vi "advent_4._bvi.vi"() -> ()   [LabVIEW 2021]
uses:
  <vilib>/Utility/file.llb/Read Delimited Spreadsheet (string).vi
  <vilib>/Utility/file.llb/Read Delimited Spreadsheet (I64).vi
panel:
  out "Array 3":i32[](array[numeric])
  out "array w/ subset deleted":string[][](array[string])
  out "all rows 2":string[][](array[string])
  out "final value":i32
  out "last number called":u8
  out "sum of unmarked":i32
  out "all rows":string[](array[string])
  out "size(s)":i32
  out "final bingo call":i32
  out "Book Number":i32
  out "Array":bool[][][](array[boolean])
  out "card values":i32[][](array[numeric])
  out "card":bool[][](array[boolean])
  out "initialized array":bool[][][](array[boolean])
  out "Array 2":i32[][][](array[numeric])
  out "subarray":string[](array[string])
  out "first row":i64[](array[numeric])
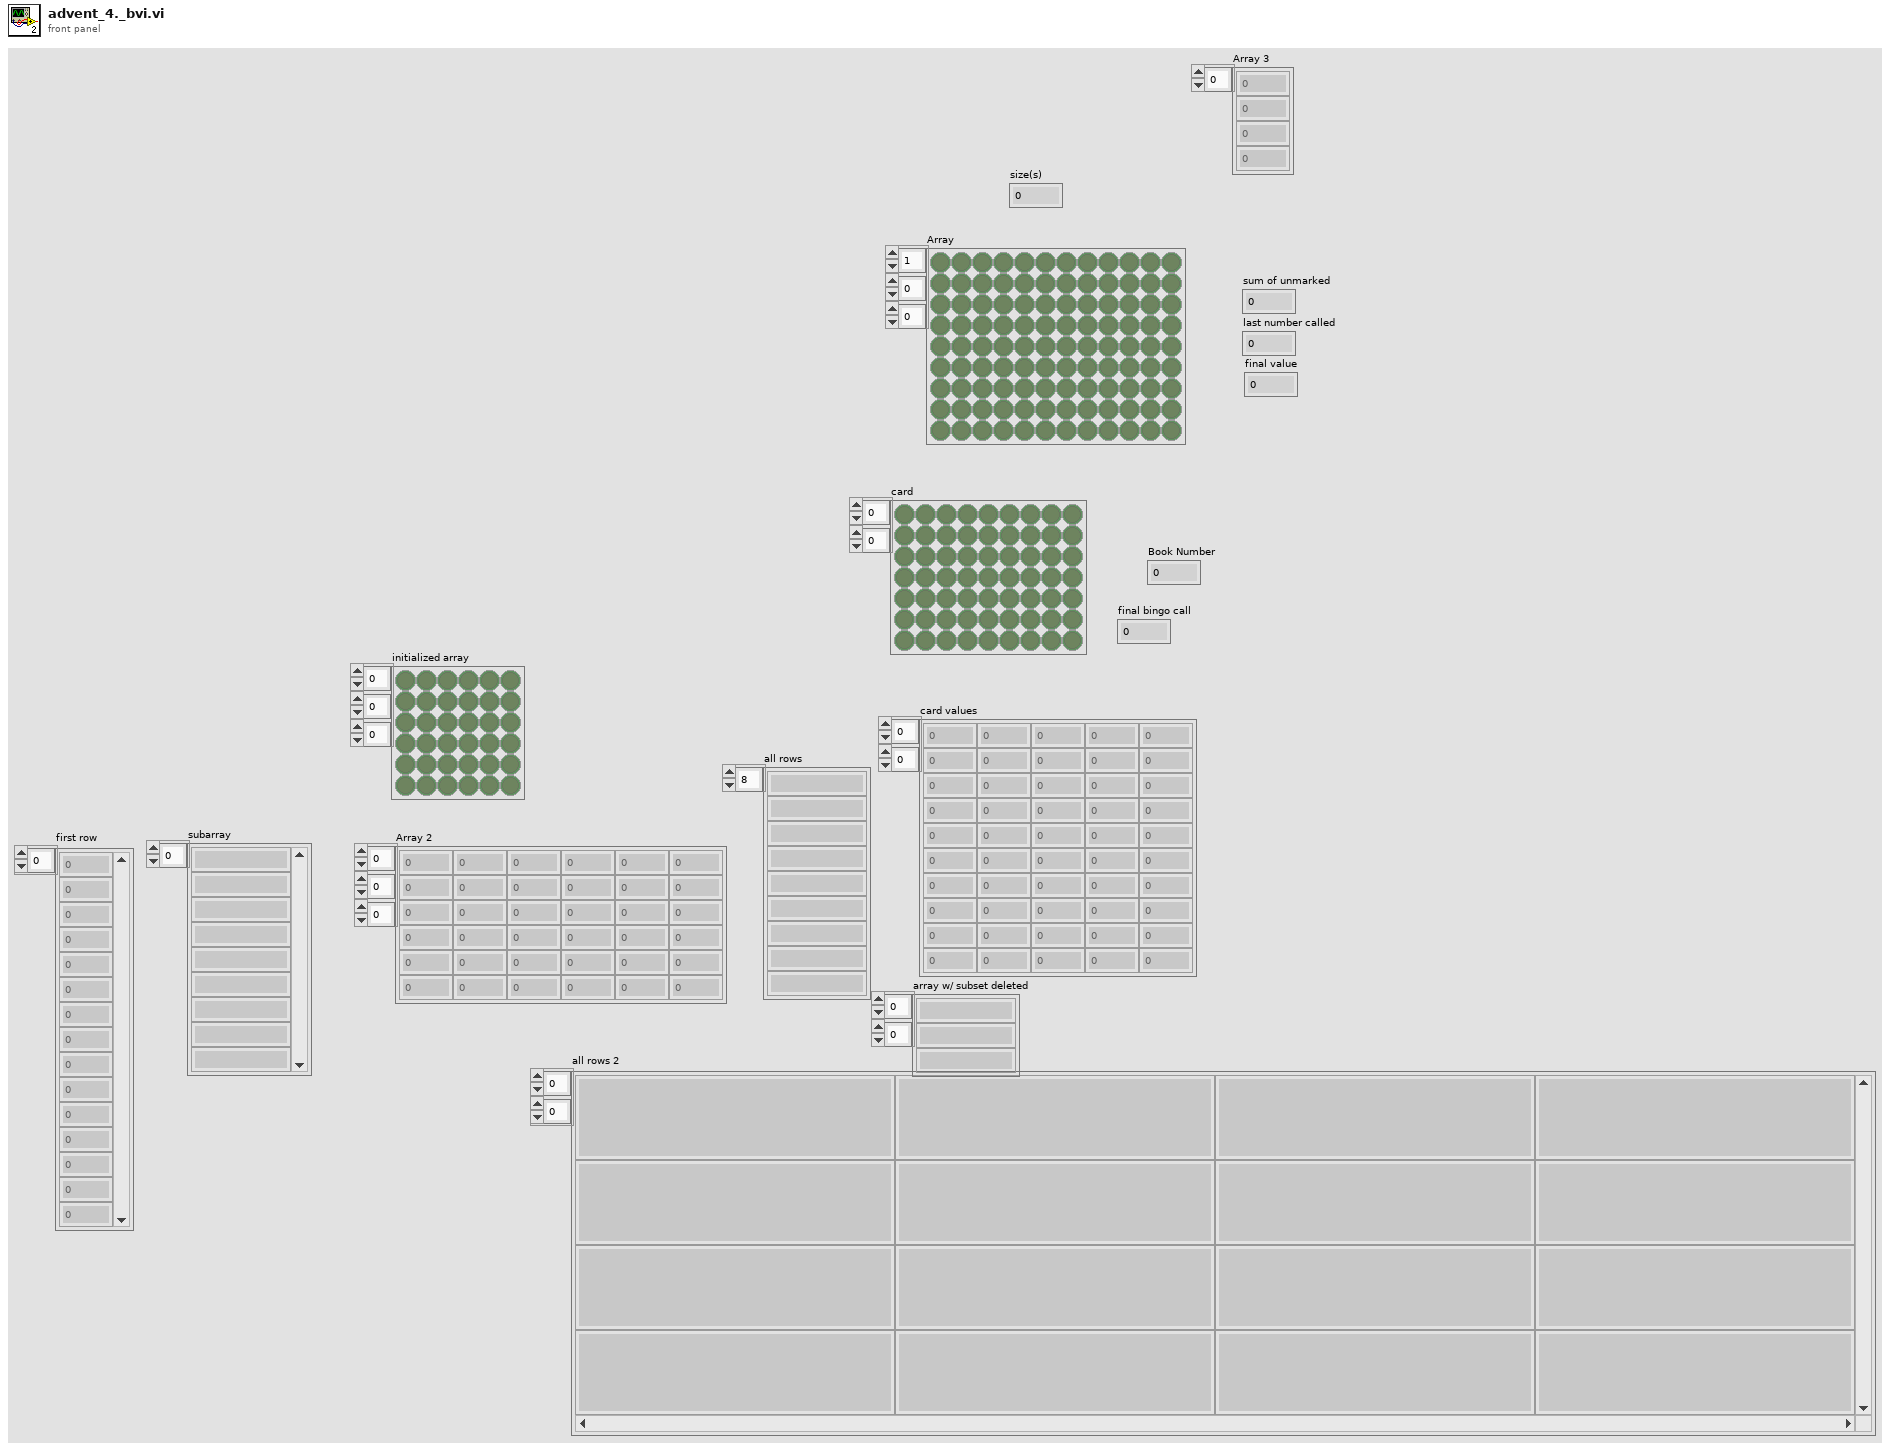
[diagram p1: front panel]
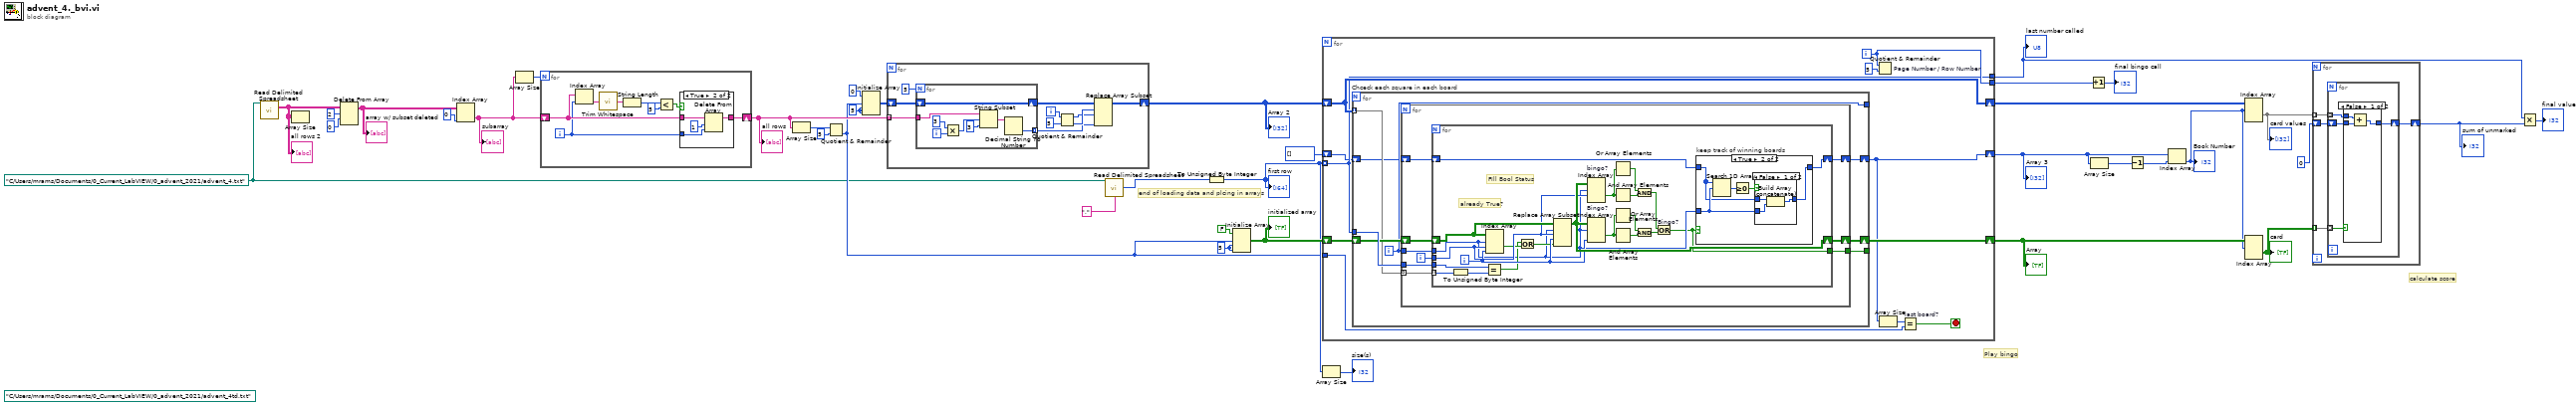
[diagram p0: block diagram]
diagram:
  w1 = path "C:/Users/mrams/Documents/0_Current_LabVIEW/0_advent_2021/advent_4.txt" ("file path (dialog if empty)")
  w25 = 5 ("dimension size")
  w26 = 5 ("dimension size")
  (unwired) path "C:/Users/mrams/Documents/0_Current_LabVIEW/0_advent_2021/advent_4td.txt" ("file path (dialog if empty)")
  # "end of loading data and plcing in arrays"
  # "calculate score"
  # "Play bingo"
  n1 = call-poly <vilib>:"Read Delimited Spreadsheet.vi"("file path (dialog if empty)"=w1) -> ("all rows"=w8:string[][])  [unwired: 9 in, 5 out]
  "all rows 2" <- w8
  n2 = Array Size(array=w8) -> ()  [unwired: 1 out]
  n3 = Delete From Array(array=w8, length=2, index (row)=0) -> (array with subset deleted=w35:string[][])  [unwired: 1 in, 1 out]
  "array w/ subset deleted" <- w35
  n4 = Index Array(array=w35, index (col)=0 ("disabled index (col)")) -> (element=w28:string[])  [unwired: 1 in]
  "subarray" <- w28
  n5 = Array Size(array=w28) -> (size(s)=w27:i32)
  n6 = for {
    N: w27 -> [_]
    shift-right: [w39] -> w31
    shift-left: w28 -> [w46]
    i -> [w45]
    n7 = Index Array(array=w46, index=w45) -> (element=w44:string)
    n8 = call <vilib>:"Trim Whitespace.vi"("string"=w44) -> ("trimmed string"=w43:string)  [unwired: 1 in]
    n9 = String Length(string=w43) -> (length=w42:i32)
    n10 = Less?(x=w42, y=5) -> (x < y?=w40:bool)
    n11 = case shown="True" w40 {
      tunnel: w46 -> [w47 w51]
      tunnel: w45 -> [_ w50]
      tunnel: [w47 w48] -> w39
      frame False {
      }
      frame True {
        n12 = Delete From Array(array=w51, length=1, index=w50) -> (array with subset deleted=w48:string[])  [unwired: 1 out]
      }
    }
  }
  "all rows" <- w31
  n13 = Array Size(array=w31) -> (size(s)=w30:i32)
  n14 = Quotient & Remainder(x=w30, y=5) -> (floor(x/y)=w3:i32)  [unwired: 1 out]
  n15 = Initialize Array(u8 0, w3, w26, w26) -> (w32:u8[][][])
  n16 = for {
    tunnel: w31 -> [w61] mode=indexing
    shift-right: [w58] -> w22
    shift-left: w32 -> [w60]
    i -> [w56]
    n17 = for {
      N: 5 -> [_]
      tunnel: w61 -> [w69]
      tunnel: [w65] -> w52 mode=indexing
      shift-right: [w64] -> w59
      shift-left: w60 -> [w64]
      i -> [w63]
      n18 = Multiply(x=3, y=w63) -> (x*y=w62:i32)
      n19 = String Subset(string=w69, offset (0)=w62, length (rest)=3 ("length (rest)")) -> (substring=w66:string)
      n20 = Decimal String To Number(string=w66) -> (number=w65:i32)  [unwired: 2 in, 1 out]
    }
    n21 = Quotient & Remainder(x=w56, y=5) -> (x-y*floor(x/y)=w53:i32, floor(x/y)=w54:i32)
    n22 = Replace Array Subset(array=w59, new element=w52, index (dim 0)=w54, index (dim 1)=w53) -> (w58:u8[][][])  [unwired: 1 in]
  }
  "Array 2" <- w22
  n23 = call-poly <vilib>:"Read Delimited Spreadsheet.vi"("file path (dialog if empty)"=w1, "delimiter (\\t)"="," ("delimiter (\\t)")) -> ("first row"=w18:i64[])  [unwired: 8 in, 5 out]
  n24 = To Unsigned Byte Integer(number=w18) -> (unsigned 8bit integer=w15:u8[])
  "first row" <- w15
  n25 = Initialize Array(FALSE, w3, w25, w25) -> (w23:bool[][][])
  "initialized array" <- w23
  n26 = for {
    tunnel: w15 -> [w75] mode=indexing
    shift-right: [w78] -> w21
    shift-left: w23 -> [w80]
    shift-right: [w77] -> w20
    shift-left: w22 -> [w77]
    tunnel: [w76] -> w19
    tunnel: [w75] -> w10
    shift-right: [w71] -> w5
    shift-left: i32[] [] -> [w72]
    tunnel: w3 -> [w73]
    i -> [w76]
    stop <- w70 stop-if-true
    n27 = for "Chceck each square in each board" {
      tunnel: w75 -> [w88]
      tunnel: w77 -> [w86] mode=indexing
      shift-right: [w85] -> w78
      shift-left: w80 -> [w87]
      tunnel: [w82] -> _
      tunnel: [w84] -> _
      shift-right: [w81] -> w71
      shift-left: w72 -> [w83]
      i -> [w84]
      n28 = for {
        tunnel: w88 -> [w95]
        tunnel: w86 -> [w96] mode=indexing
        shift-right: [w93] -> w85
        shift-left: w87 -> [w97]
        tunnel: w84 -> [w94]
        tunnel: [w90] -> w82
        shift-right: [w89] -> w81
        shift-left: w83 -> [w91]
        i -> [w92]
        n29 = for {
          tunnel: w96 -> [w118] mode=indexing
          tunnel: w95 -> [w119]
          shift-right: [w117] -> w93
          shift-left: w97 -> [w107]
          tunnel: w94 -> [w101]
          tunnel: w92 -> [w106]
          tunnel: [w98] -> w90
          shift-right: [w99] -> w89
          shift-left: w91 -> [w100]
          i -> [w105]
          # "FIll Bool Status"
          # "already True?"
          n30 = To Unsigned Byte Integer(number=w118) -> (unsigned 8bit integer=w108:u8)
          n31 = Equal?(x=w119, y=w108) -> (x = y?=w103:bool)
          n32 = Index Array(array=w107, index (dim 0)=w101, index (dim 1)=w106, index (dim 2)=w105) -> (element=w104:bool)
          n33 = Or(x=w103, y=w104) -> (x .or. y?=w102:bool)
          n34 = Replace Array Subset(array=w107, new element=w102, index (dim 0)=w101, index (dim 1)=w106, index (dim 2)=w105) -> (w117:bool[][][])
          n35 = Index Array "bingo?"(array=w117, index (dim 0)=w101, index (dim 1)=w106) -> (element=w116:bool[])  [unwired: 1 in]
          n36 = Index Array "Bingo?"(array=w117, index (dim 0)=w101, index (dim 2)=w105) -> (element=w115:bool[])  [unwired: 1 in]
          n37 = Or Array Elements(Boolean array=w116) -> (logical OR=w114:bool)
          n38 = And Array Elements(Boolean array=w116) -> (logical AND=w113:bool)
          n39 = Or Array Elements(Boolean array=w115) -> (logical OR=w112:bool)
          n40 = And Array Elements(Boolean array=w115) -> (logical AND=w111:bool)
          n41 = And(x=w114, y=w113) -> (x .and. y?=w109:bool)
          n42 = And(x=w112, y=w111) -> (x .and. y?=w110:bool)
          n43 = Or "Bingo?"(x=w109, y=w110) -> (x .or. y?=w98:bool)
          n44 = case "keep track of winning boards" shown="True" w98 {
            tunnel: w100 -> [w120 w124]
            tunnel: [w120 w123] -> w99
            tunnel: w101 -> [_ w125]
            frame False {
            }
            frame True {
              n45 = Search 1D Array(1D array=w124, element=w125) -> (index of element=w122:i32)  [unwired: 1 in]
              n46 = Greater Or Equal To 0?(x=w122) -> (x >= 0?=w121:bool)
              n47 = case shown="False" w121 {
                tunnel: w124 -> [w128 w129]
                tunnel: w125 -> [w127 _]
                tunnel: [w126 w129] -> w123
                frame False {
                  n48 = Build Array (concatenate)(w128, w127) -> (w126:i32[])
                }
                frame True {
                }
              }
            }
          }
        }
      }
    }
    n49 = Quotient & Remainder "Page Number / Row Number"(x=w76, y=5) -> ()  [unwired: 2 out]
    n50 = Array Size(array=w71) -> (size(s)=w74:i32)
    n51 = Equal? "last board?"(x=w74, y=w73) -> (x = y?=w70:bool)
  }
  "Array" <- w21
  "last number called" <- w10
  "Array 3" <- w5
  n52 = Array Size(array=w15) -> (size(s)=→"size(s)":i32)
  n53 = Increment(x=w19) -> (x+1=→"final bingo call":i32)
  n54 = Array Size(array=w5) -> (size(s)=w7:i32)
  n55 = Decrement(x=w7) -> (x-1=w6:i32)
  n56 = Index Array(array=w5, index=w6) -> (element=w4:i32)
  "Book Number" <- w4
  n57 = Index Array(array=w20, index (dim 0)=w4) -> (element=w13:u8[][])  [unwired: 2 in]
  "card values" <- w13
  n58 = Index Array(array=w21, index (dim 0)=w4) -> (element=w14:bool[][])  [unwired: 2 in]
  "card" <- w14
  n59 = for {
    tunnel: w14 -> [w133] mode=indexing
    tunnel: w13 -> [w132] mode=indexing
    shift-right: [w130] -> w11
    shift-left: 0 -> [w131]
    n60 = for {
      tunnel: w133 -> [w137] mode=indexing
      tunnel: w132 -> [w136] mode=indexing
      shift-right: [w134] -> w130
      shift-left: w131 -> [w135]
      n61 = case shown="False" w137 {
        tunnel: w136 -> [w140 _]
        tunnel: w135 -> [w139 w141]
        tunnel: [w138 w141] -> w134
        frame False {
          n62 = Add(x=w140, y=w139) -> (x+y=w138:i32)
        }
        frame True {
        }
      }
    }
  }
  "sum of unmarked" <- w11
  n63 = Multiply(x=w10, y=w11) -> (x*y=→"final value":i32)
